vi "KeithleyVoltage.vi"(8 "error in":errorcluster, 9 "channel (6)":i32=6, 10 "address (16)":i16, 11 "bus":i32) -> (0 "error out":errorcluster, 3 "Voltage":dbl)   [LabVIEW 2017]
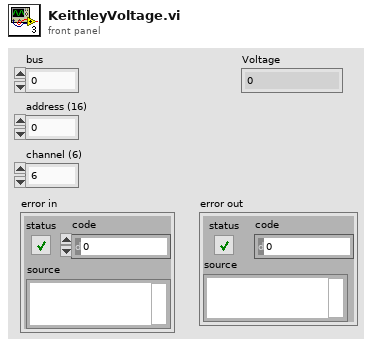
[diagram p1: front panel]
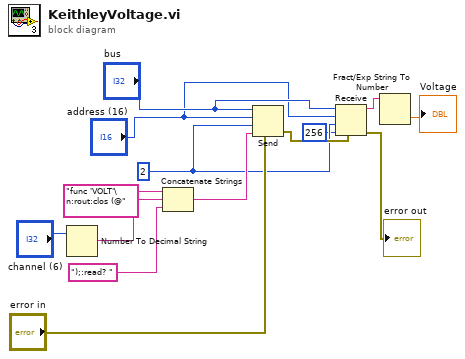
[diagram p0: block diagram]
diagram:
  w5 = i16 2 ("mode")
  n1 = Number To Decimal String(number="channel (6)") -> (decimal integer string=w13:string)  [unwired: 1 in]
  n2 = Concatenate Strings("func 'VOLT'\n:rout:clos (@", w13, ");:read? ") -> (w10:string)
  n3 = Send(0:"bus", 2:"address (16)", 3:w5, 4:"error in", 5:w10) -> (8:w9:errorcluster)  [unwired: 2 out]
  n4 = Receive(4:w9, 6:256 ("count"), 7:w5, 8:"address (16)", 9:"bus") -> (0:→"error out":errorcluster, 3:w2:string)  [unwired: 2 out]
  n5 = Fract/Exp String To Number(string=w2) -> (number=→"Voltage":dbl)  [unwired: 3 in, 1 out]
